vi "Process.vi"(9 "process sync":refnum<notifier>, 11 "Log_Engine in":refnum<class "Log_Engine.lvclass">) -> ()   [LabVIEW 2019, in "Log_Engine.lvclass"]
doc: "Developed by Kevin Thompson\nkevin@thompsonengineering.net\n\nCopyright 2018\nThompson Engineering, LLC"
uses:
  Log_Engine.lvclass
  DataTypes/Read Data--cluster.ctl
  DataTypes/AsynCmd_Log_Engine--enum.ctl
  DataTypes/Process - AppData--cluster.ctl
  DataTypes/Settings--cluster.ctl
  DataTypes/Dependency--cluster.ctl
  Config/Config.lvclass
  DAQ_Engine/DAQ_Engine.lvclass
  DataTypes/Public Events--cluster.ctl
  Common/DataTypes/TD Async CmdMsg EventData--cluster.ctl
  DataTypes/LogStateChg EvData--cluster.ctl
  DataTypes/LogStateEvData--cluster.ctl
  Common/DataTypes/LogState--enum.ctl
  DataTypes/TDMSStateChg EvData--cluster.ctl
  DataTypes/TDMSStateEvData--cluster.ctl
  Common/DataTypes/TDMSState--enum.ctl
  Common/DataTypes/InverterWaveforms--QRef.ctl
  Common/DataTypes/InverterWaveforms--cluster.ctl
  Common/DataTypes/ChannelWaveforms--cluster.ctl
  DataTypes/WriteLoopPvtData--Cluster.ctl
  Log_Engine.lvclass/Log_Engine.ctl
  DAQ_Engine/DAQ_Engine.lvclass/DAQ_Engine.ctl
  Accessors/Get Settings.vi
  Accessors/Get PublicEvents.vi
  Accessors/Get Dependency.vi
  Accessors/Get InvWfmsQRef.vi
  <vilib>/TELLC/SMQ/Add States to Queue using MultiLine String with vData.vi
  <userlib>/_OpenG.lib/file/file.llb/File Exists - Scalar__ogtk.vi
  <vilib>/Utility/file.llb/Write Delimited Spreadsheet (string).vi
panel:
  out "Log_Engine ReadData":T1
  in  "Exit":bool
  # "local data monitoring"
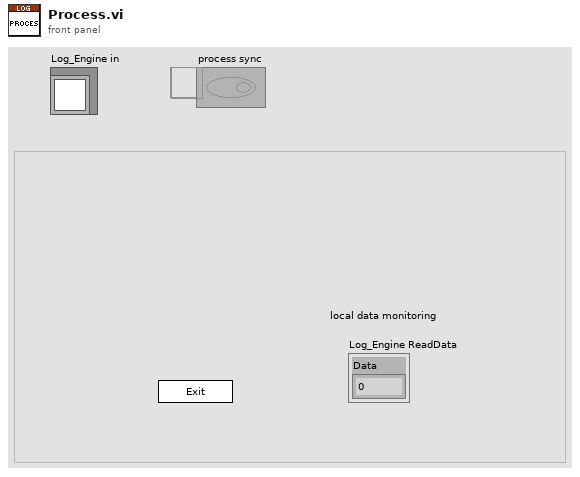
[diagram p1: front panel]
types:
  T1 = typedef "Log_Engine.lvclass/Read Data--cluster.ctl" = cluster{"Data":dbl}
  T2 = typedef "Log_Engine.lvclass/AsynCmd_Log_Engine--enum.ctl" = enum16{"Log_Engine.StartLog", "Log_Engine.StopLog", "Log_Engine.StartESRLog", "Log_Engine.StopESRLog"}
  T3 = typedef "InverterWaveforms--QRef.ctl" = refnum<queue>
  T4 = typedef "InverterWaveforms--cluster.ctl" = cluster{"Phase1 ChanWfms":T5, "Phase2 ChanWfms":T5, "Phase3 ChanWfms":T5}
  T5 = typedef "ChannelWaveforms--cluster.ctl" = cluster{"Iin ripple ":waveform(dbl), "Iout ripple ":waveform(dbl), "Vout 60Hz":waveform(dbl), "Iout 60Hz":waveform(dbl)}
  T6 = typedef "TD MeasData--cluster.ctl" = cluster{"Timestamp":timestamp, "ESR_Ohm":dbl[], "DUT data":T7[], "DUT INVERTER data":cluster{"Raw ESR sum":dbl, "scaled raw ESR sum":dbl, "scaled and averaged raw ESR sum":dbl, "Total power":dbl}[]}
  T7 = typedef "InverterPhaseData--cluster.ctl" = cluster{"RawESR_Ohm":dbl, "TcompAvgESR_Ohm":dbl, "VoutRMS_V":dbl, "IoutRMS_A":dbl, "PF":dbl, "AvgPF":dbl, "Power_W":dbl, "AvgPower_W":dbl, "efficiency":dbl}
  T8 = typedef "Log_Engine.lvclass/Process - AppData--cluster.ctl" = cluster{"Core":cluster{"Current VI Reference":refnum<vi>, "Close Panel on Exit?":bool}, "Your Boolean data":bool, "Your string data":string, "SMQ":refnum<queue>, "Self Reference":refnum<class "Log_Engine.lvclass">, "Simulation?":bool, "process sync":refnum<notifier>, "vData":variant, "Settings":T9, "Dependency":T10, "Public Events":T11, "InverterWaveformsQ":T3, "FileHandle":T12, "Initialized?":bool, "LogState":T13, "TDMSState":T14, "CSV BaseFN":string[], "TDMS BaseFN":string[], "TDMS_Folder":path, "CSV_Folder":path}
  T9 = typedef "Log_Engine.lvclass/Settings--cluster.ctl" = cluster{"Simulation":bool, "TDMS_FolderPath":string, "CSV_FolderPath":string, "TDMS_FileName_Prefix":string, "CSV_FileName_Prefix":string, "TDMS_LogDuration(s)":dbl, "CSV_LogDuration(s)":dbl}
  T10 = typedef "Log_Engine.lvclass/Dependency--cluster.ctl" = cluster{"Config":refnum<class "Config.lvclass">, "DAQ_Engine":refnum<class "DAQ_Engine.lvclass">}
  T11 = typedef "Log_Engine.lvclass/Public Events--cluster.ctl" = cluster{"Log_Engine.AsyncCmd Event":refnum<user-event>, "Log_Engine.AsyncMsg Event":refnum<user-event>, "stop process":refnum<user-event>, "Log_Engine.LogStateChg Ev":refnum<user-event>, "Log_Engine.TDMSStateChg Ev":refnum<user-event>}
  T12 = typedef "Log_Engine.lvclass/WriteLoopPvtData--Cluster.ctl" = cluster{"CSV File Path":path[], "CSV_Initialized":bool, "tdms file ref":refnum<k34>[], "tdms_Initialized":bool, "TDMS File Start Time":dbl, "CSV File Start Time":dbl, "TDMSFileCounter":u32, "CSVFileCounter":u32}
  T13 = typedef "LogState--enum.ctl" = enum16{"Unknown", "Stopped", "Running", "Error"}
  T14 = typedef "TDMSState--enum.ctl" = enum16{"Unknown", "Stopped", "Running", "Error"}
  T15 = enum16{"open", "open or create", "create or replace", "create", "open (read-only)"}
  T16 = enum16{"open", "replace", "create", "open or create", "replace or create", "replace or create with confirmation"}
  T17 = typedef "TD Pathnames--cluster.ctl" = cluster{"RunTimeSys?":bool, "AppFolder":path, "ExecutablePath":path, "ConfigFolder":path, "DataLogFolder":path, "SystemLogFolder":path, "SeqFolder":path, "MainStartupPathname":path, "MainUIPathname":path, "SystemEventsFile":path, "SeqEventsFile":path, "Config SettingsFile":path, "DAQ IOConfigFile":path, "SystemSimulation":bool}
  T18 = typedef "InverterWaveforms--cluster.ctl" = T5[]
  T19 = enum32{"invalid app kind", "Development System", "Run Time System", "Student Edition", "Embedded LabVIEW", "Evaluation", "Custom"}
  T20 = enum32{"Invalid", "Standard", "Closed", "Hidden", "Minimized", "Maximized"}
  T21 = typedef "DAQ_Engine.lvclass/DAQStateEvData--cluster.ctl" = cluster{"DAQState":T22, "vData":variant}
  T22 = typedef "DAQState--enum.ctl" = enum16{"Unknown", "Stopped", "Running", "Error"}
  T23 = cluster{"Current VI Reference":refnum<vi>, "Close Panel on Exit?":bool}
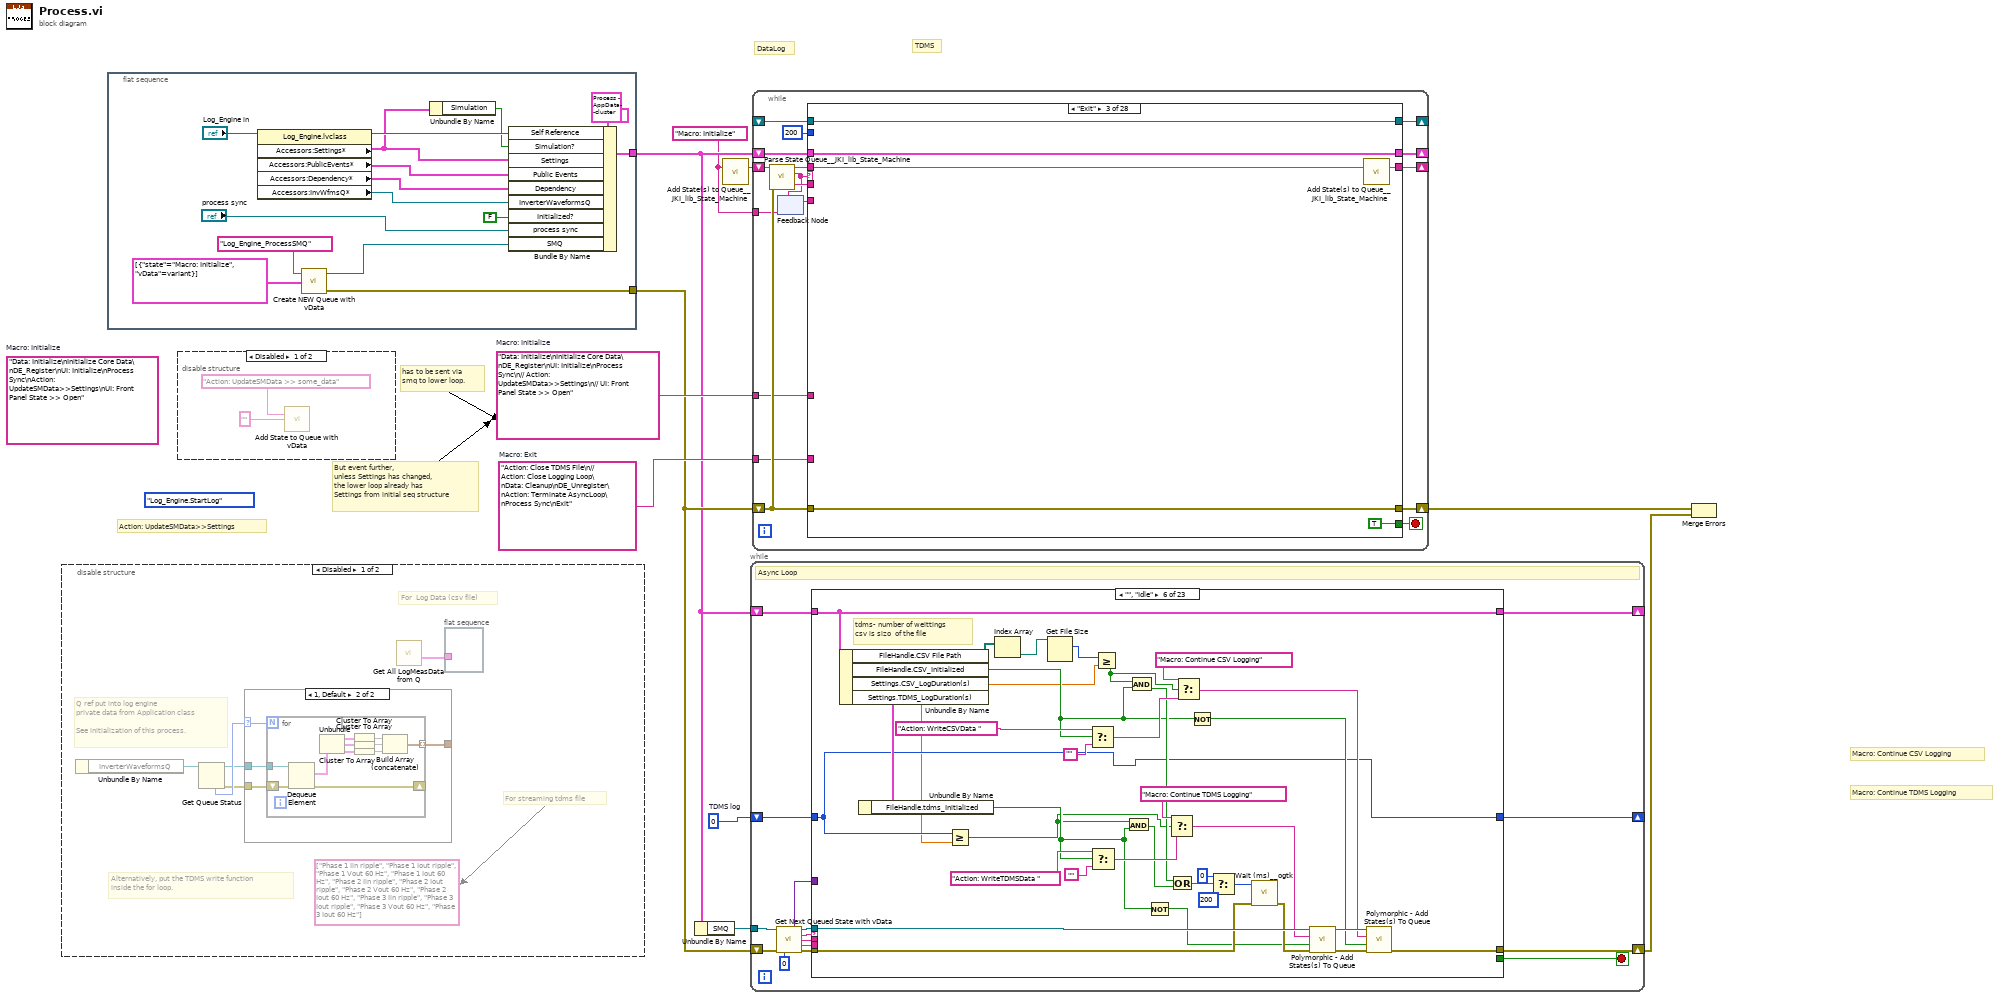
[diagram p0: block diagram]
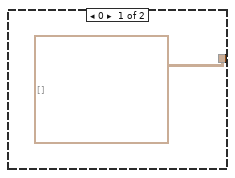
[diagram p2: hidden frame]
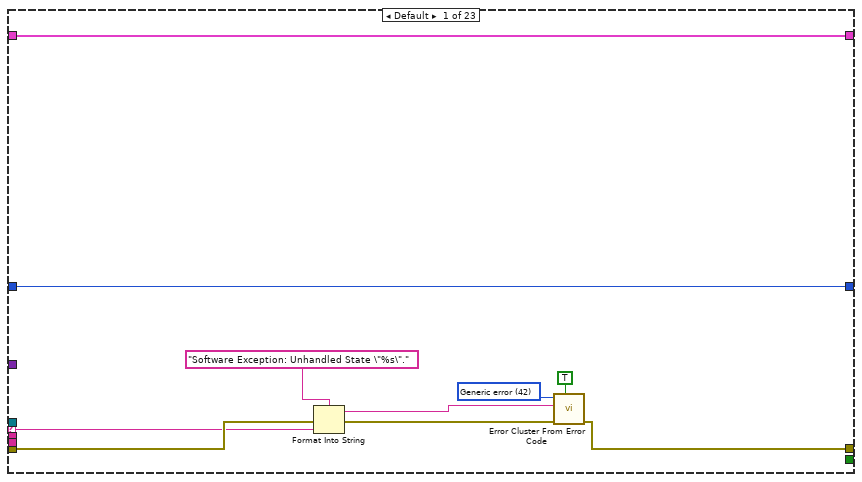
[diagram p5: hidden frame]
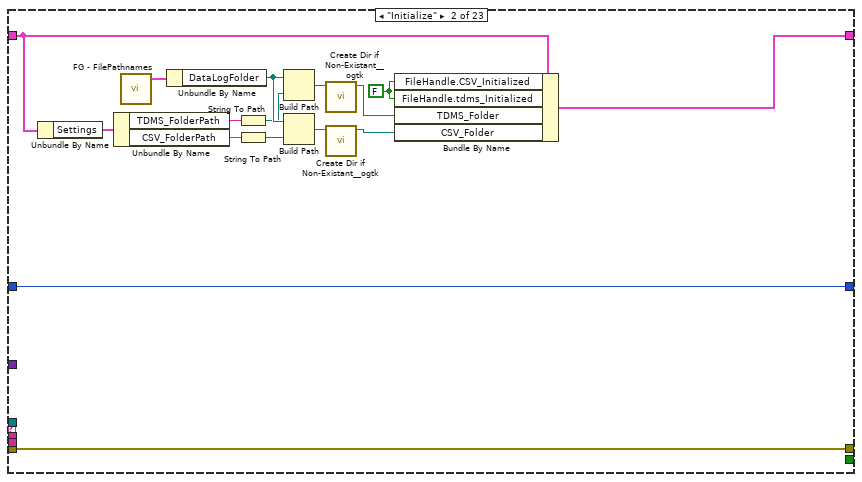
[diagram p6: hidden frame]
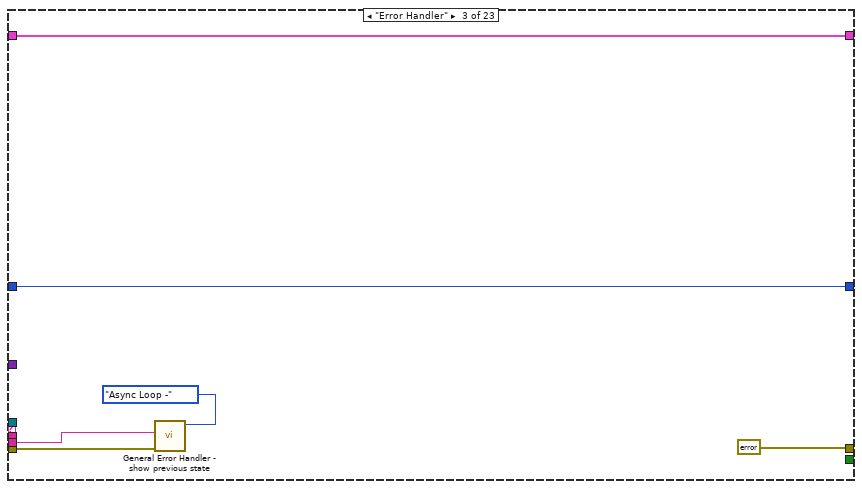
[diagram p7: hidden frame]
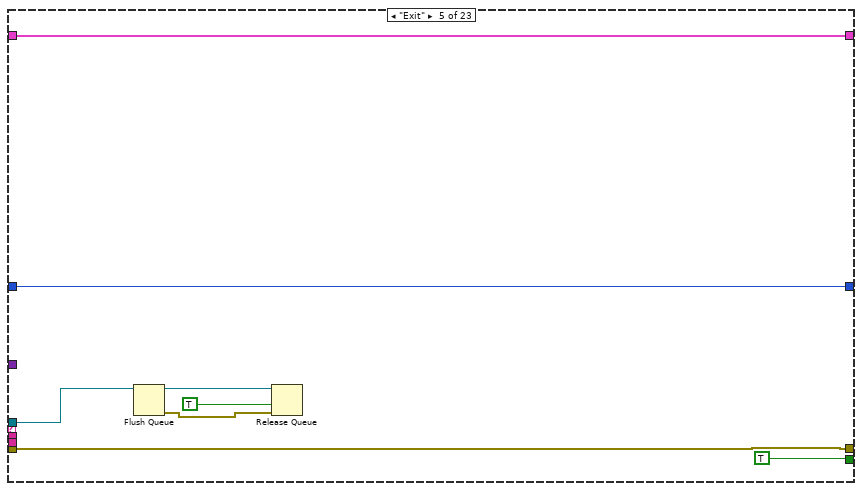
[diagram p9: hidden frame]
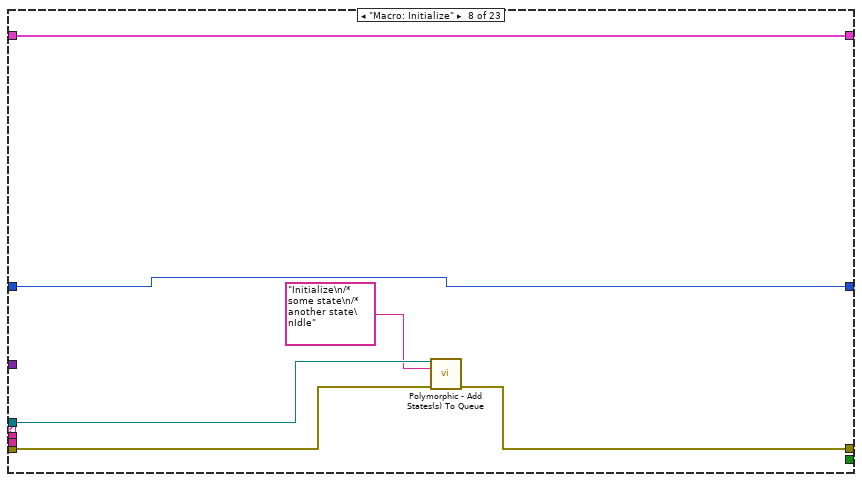
[diagram p11: hidden frame]
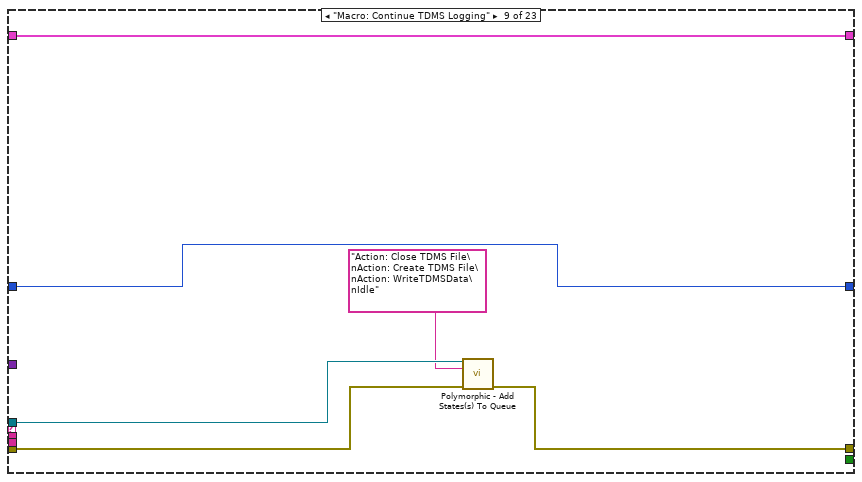
[diagram p12: hidden frame]
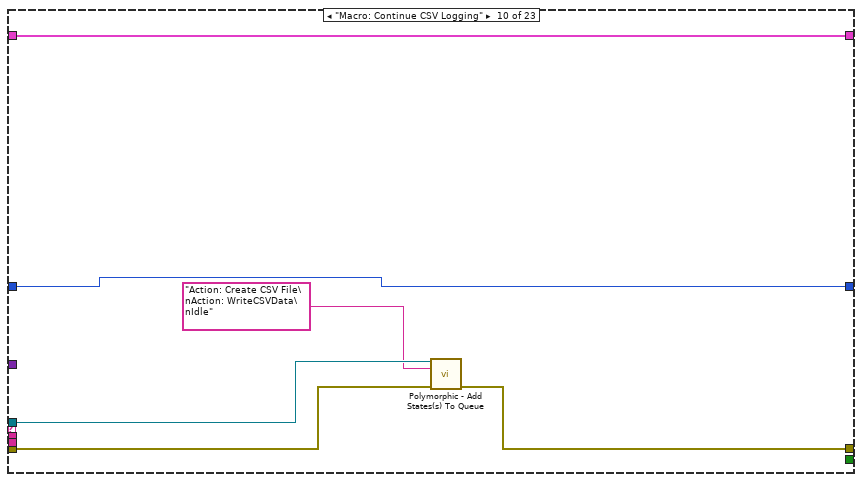
[diagram p13: hidden frame]
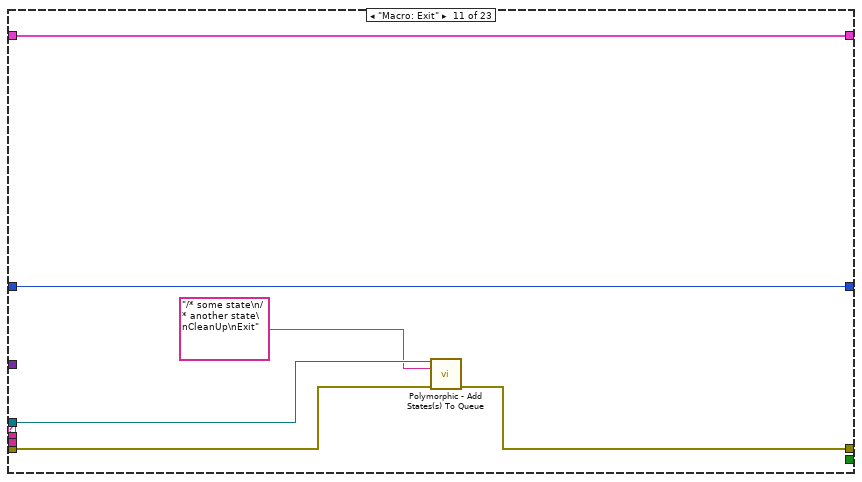
[diagram p14: hidden frame]
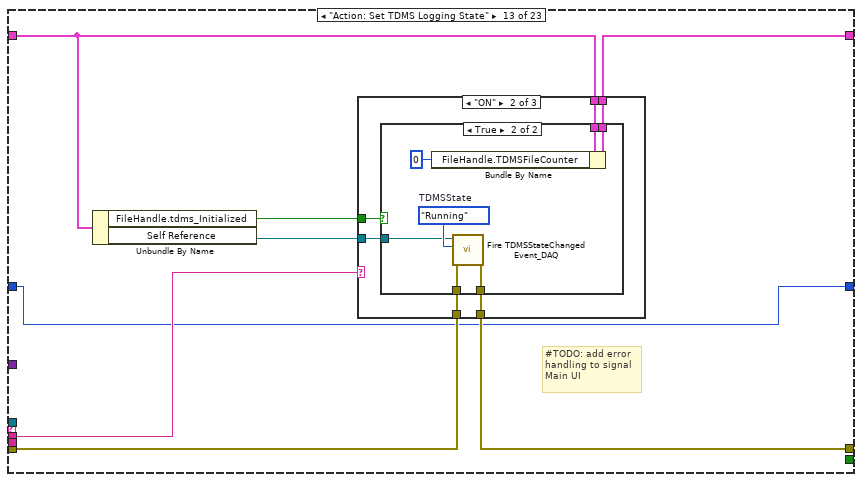
[diagram p16: hidden frame]
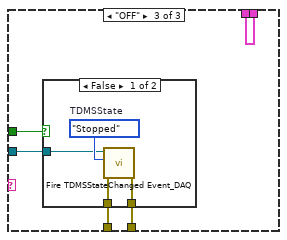
[diagram p19: hidden frame]
diagram:
  w1 = 0  # TDMS log
  (unwired) "Data: Initialize\nInitialize Core Data\nDE_Register\nUI: Initialize\nProcess Sync\nAction: UpdateSMData>>Settings\nUI: Front Panel State >> Open"  # Macro: Initialize
  (unwired) AsynCmd_Log_Engine--enum."Log_Engine.StartLog" ("AsyncCmd")
  w8 = "Action: Close TDMS File\n// Action: Close Logging Loop\nData: Cleanup\nDE_Unregister\nAction: Terminate AsyncLoop\nProcess Sync\nExit"  # Macro: Exit
  w9 = "Data: Initialize\nInitialize Core Data\nDE_Register\nUI: Initialize\nProcess Sync\n// Action: UpdateSMData>>Settings\n// UI: Front Panel State >> Open"  # Macro: Initialize
  w2 = "Macro: Initialize"
  # "TDMS"
  # "DataLog"
  # "Macro: Continue TDMS Logging"
  # "Macro: Continue CSV Logging"
  # "But event further,\nunless Settings has changed,\nthe lower loop already has\nSettings from initial seq structure"
  # "has to be sent via\nsmq to lower loop."
  # "Action: UpdateSMData>>Settings"
  n1 = disable-structure shown="Disabled" {
    frame Disabled {
      (unwired) string[] ["Phase 1 Iin ripple", "Phase 1 Iout ripple", "Phase 1 Vout 60 Hz", "Phase 1 Iout 60 Hz", "Phase 2 Iin ripple", "Phase 2 Iout ripple", "Phase 2 Vout 60 Hz", "Phase 2 Iout 60 Hz", "Phase 3 Iin ripple", "Phase 3 Iout ripple", "Phase 3 Vout 60 Hz", "Phase 3 Iout 60 Hz"] ("channel name(s) in (Untitled)")
      # "Q ref put into log engine\nprivate data from Application class\n\nSee initialization of this process."
      # "Alternatively, put the TDMS write function\ninside the for loop."
      # "For streaming tdms file"
      # "For  Log Data (csv file)"
      n2 = Unbundle By Name() -> ("InverterWaveformsQ"=w11:T3)  [unwired: 1 in]
      n3 = Get Queue Status(queue=w11) -> (queue out=w14:T3, error out=w13:errorcluster, # elements in queue=w15:i32)  [unwired: 2 in, 5 out]
      n4 = case shown="1, Default" w15 {
        selector: w15 -> [_ w20]
        tunnel: w14 -> [_ w19]
        tunnel: w13 -> [_ w18]
        tunnel: [waveform(dbl)[][] [] w17] -> _
        frame 0 {
        }
        frame 1, Default {
          n5 = for {
            N: w20 -> [_]
            tunnel: w19 -> [w31]
            shift-right: [w29] -> _
            shift-left: w18 -> [w30]
            tunnel: [w21] -> w17 mode=indexing
            n6 = Dequeue Element(queue=w31, error in (no error)=w30) -> (element=w28:T4, error out=w29:errorcluster)  [unwired: 1 in, 2 out]
            n7 = Unbundle(w28) -> ("Phase1 ChanWfms"=w27:T5, "Phase2 ChanWfms"=w26:T5, "Phase3 ChanWfms"=w25:T5)
            n8 = Cluster To Array(cluster=w27) -> (array=w24:waveform(dbl)[])
            n9 = Cluster To Array(cluster=w26) -> (array=w23:waveform(dbl)[])
            n10 = Cluster To Array(cluster=w25) -> (array=w22:waveform(dbl)[])
            n11 = Build Array (concatenate)(w24, w23, w22) -> (w21:waveform(dbl)[])
          }
        }
      }
      n12 = call "Get All LogMeasData from Q.vi"() -> ("MeasData[] out"=w12:T6[])  [unwired: 8 in, 3 out]
      n13 = flat-sequence {
        tunnel: w12 -> [_]
        frame #0 {
        }
      }
    }
    frame Enabled {
    }
  }
  n14 = flat-sequence {
    tunnel: [w46] -> w5
    tunnel: [w43] -> w7
    frame #0 {
      n15 = property class="Log_Engine.lvclass"(reference="Log_Engine in") -> (reference out=w40:refnum<class "Log_Engine.lvclass">, "Accessors:Settings*"=w32:T9, "Accessors:PublicEvents*"=w37:T11, "Accessors:Dependency*"=w38:T10, "Accessors:InvWfmsQ*"=w34:T3)  [unwired: 1 in, 1 out]
      n16 = call <vilib>:"Create NEW Queue with vData.vi"("Initial States"=cluster{"state":string, "vData":variant}[] [{"state"="Macro: Initialize", "vData"=variant}], "Name (SMQ)"="Log_Engine_ProcessSMQ") -> ("error out"=w43:errorcluster, "queue out"=w45:refnum<queue>)  [unwired: 2 in]
      n17 = Unbundle By Name(w32) -> ("Simulation"=w33:bool)
      n18 = Bundle By Name(cluster=T8 {"Core"={"Current VI Reference"=refnum, "Close Panel on Exit?"=FALSE}, "Your Boolean data"=FALSE, "Your string data"="", "SMQ"=refnum, "Self Reference"=refnum, "Simulation?"=FALSE, "process sync"=refnum, "vData"=variant, "Settings"={"Simulation"=FALSE, "TDMS_FolderPath"="", "CSV_FolderPath"="", "TDMS_FileName_Prefix"="", "CSV_FileName_Prefix"="", "TDMS_LogDuration(s)"=0.0, "CSV_LogDuration(s)"=0.0}, "Dependency"={"Config"=refnum, "DAQ_Engine"=refnum}, "Public Events"={"Log_Engine.AsyncCmd Event"=refnum, "Log_Engine.AsyncMsg Event"=refnum, "stop process"=refnum, "Log_Engine.LogStateChg Ev"=refnum, "Log_Engine.TDMSStateChg Ev"=refnum}, "InverterWaveformsQ"=refnum, "FileHandle"={"CSV File Path"=[], "CSV_Initialized"=FALSE, "tdms file ref"=[], "tdms_Initialized"=FALSE, "TDMS File Start Time"=0.0, "CSV File Start Time"=0.0, "TDMSFileCounter"=0, "CSVFileCounter"=0}, "Initialized?"=FALSE, "LogState"=enum."Unknown", "TDMSState"=enum."Unknown", "CSV BaseFN"=[], "TDMS BaseFN"=[], "TDMS_Folder"=path "", "CSV_Folder"=path ""} ("SM2 AppData"), "Self Reference"=w40, "Simulation?"=w33, "Settings"=w32, "Public Events"=w37, "Dependency"=w38, "InverterWaveformsQ"=w34, "Initialized?"=FALSE, "process sync"="process sync", "SMQ"=w45) -> (w46:T8)
    }
  }
  n19 = disable-structure shown="Disabled" {
    frame Disabled {
      n20 = call <vilib>:"Add State to Queue with vData.vi"("state in"="Action: UpdateSMData >> some_data", "vData (\"\")"="") -> ()  [unwired: 10 in, 4 out]
    }
    frame Enabled {
    }
  }
  n21 = Unbundle By Name(w5) -> ("SMQ"=w6:refnum<queue>)
  n22 = call <vilib>:"Add State(s) to Queue__JKI_lib_State_Machine.vi"("State(s) in (\"\")"=w2) -> ("States Out"=w10:string)  [unwired: 14 in]
  n23 = while {
    shift-right: [w60] -> w3
    shift-left: w7 -> [w62]
    tunnel: w6 -> [w58]
    shift-right: [w56] -> _
    shift-left: w5 -> [w57]
    shift-right: [w50] -> _
    shift-left: w1 -> [w49]
    stop <- w51 stop-if-true
    # "Async Loop"
    n24 = call <vilib>:"Get Next Queued State with vData.vi"("queue in"=w58, "error in (no error)"=w62, "timeout (100)"=0) -> ("vData out"=w55:variant, "queue out"=w59:refnum<queue>, "Next State"=w63:string, "queued msg"=w53:string, "Prev State"=w52:string, "error out"=w61:errorcluster)  [unwired: 6 in, 1 out]
    n25 = case shown="\"\", \"Idle\"" w63 {
      tunnel: w59 -> [_ _ _ _ w100 w134 _ w149 w155 w161 w167 _ _ _ _ _ _ _ _ _ _ _ w398]
      tunnel: w53 -> [_ _ _ _ _ _ _ _ _ _ _ _ w178 w213 _ _ _ _ _ _ _ w386 w400]
      selector: w63 -> [w65 _ _ _ _ _ _ _ _ _ _ _ _ _ _ _ _ _ _ _ _ _ _]
      tunnel: w61 -> [w67 w89 w92 w98 w106 w126 w144 w148 w154 w160 w166 w171 w175 w210 w243 w270 w312 w343 w361 w373 w380 w385 w395]
      tunnel: [w66 w89 errorcluster {"status"=FALSE, "code"=0, "source"=""} ("error constant") w98 w106 w133 w144 w147 w153 w159 w165 w171 w176 w211 w252 w277 w314 w340 w357 w373 w379 w388 w394] -> w60
      tunnel: w57 -> [w73 w85 w95 w97 w105 w135 w143 w150 w156 w162 w168 w170 w173 w208 w256 w281 w311 w344 w359 w374 w382 w391 w397]
      tunnel: [w73 w87 w95 w97 w105 w135 w143 w150 w156 w162 w168 w170 w174 w209 w259 w287 w311 w344 w358 w376 w382 w391 w396] -> w56
      tunnel: w55 -> [_ _ _ _ _ _ _ _ _ _ _ _ _ _ _ _ _ _ _ _ _ _ w399]
      tunnel: w52 -> [_ _ w91 _ _ _ _ _ _ _ _ _ _ _ _ _ _ _ _ _ _ _ _]
      tunnel: [_ _ _ _ TRUE _ _ _ _ _ _ _ _ _ _ _ _ _ _ _ _ _ _] -> w51
      tunnel: [w64 w74 w90 w96 w99 w114 w142 w145 w151 w157 w163 w169 w172 w207 0 w276 w309 w338 w356 w372 w377 w383 w392] -> w50
      tunnel: w49 -> [w64 w74 w90 w96 w99 w114 w142 w145 w151 w157 w163 w169 w172 w207 _ w276 w310 w338 w356 w372 w377 w383 w392]
      frame Default {
        w69 = 42 items=["No error", "Argument error", "Memory is full", "Out of zone", "End of file", "File already open", "Generic file I/O error", "File not found", "File permission error", "Disk is full", "Duplicate path", "Too many files open", "System feature not enabled", "Resource file not found", "Cannot add resource", "Resource not found", "Image not found", "Image memory error", "Pen does not exist", "Config type invalid", "Config token not found", "Config parse error", "Config memory error", "Bad external code format", "Bad external code offset", "External code not present", "Null window", "Destroy window error", "Null menu", "Print aborted", "Bad print record", "Print driver error", "Windows error during printing", "Memory error during printing", "Print dialog error", "Generic print error", "Invalid device refnum", "Device not found", "Device parameter error", "Device unit error", "Cannot open device", "Device call aborted", "Generic error", "Cancelled by user", "Object ID too low", "Object ID too high", "Object not in heap", "Unknown heap", "Unknown object (invalid DefProc)", "Unknown object (DefProc not in table)", "Message out of range", "Invalid (null) method", "Unknown message", "Manager call not supported", "Bad address", "Network operation in progress", "Network operation timed out", "Connection is busy", "Network attribute not supported", "Network error", "Address in use", "System out of memory", "Connection aborted", "Connection refused", "Not connected", "Already connected", "Connection closed", "Initialization error (interapplication manager)", "Bad occurrence", "Wait on unbound occurrence handler", "Occurrence queue overflow", "Datalog type conflict", "Unused", "Unrecognized type (interapplication manager)", "Memory corrupt", "Failed to make temporary DLL", "Old CIN version", "Drag socket not found", "Failed to load drop-object", "Failed to register OLE object", "Failed to release OLE object", "Format specifier type mismatch", "Unknown format specifier", "Too few format specifiers", "Too many format specifiers", "Scan failed", "Newer CIN version", "Error converting to variant", "Runtime menu error", "Password tampered", "Variant attribute not found", "Incompatible variant data type", "Event data is not available", "Event Store is not present", "Occurrence is not found", "Event Queue is not created", "Event info is not available", "Refnum passed is NULL", "Error retrieving Class GUID", "Error retrieving CoClass GUID", "Error retrieving TypeLib GUID.", "Bad built application magic bytes.", "Specific driver is different from the specific driver associated with the Logical Name.", "There is no session opened to the class driver.", "Max Error", "MAX - Error with config objects", "MAX - Error loading configuration", "MAX - Group not supported"]
        n26 = Format Into String(format string="Software Exception: Unhandled State \"%s\"." ("message"), error in=w67, w65) -> (resulting string=w70:string, error out=w71:errorcluster)  [unwired: 1 in]
        n27 = call <vilib>:"Error Cluster From Error Code.vi"("show call chain? (False)"=TRUE, "error in (no error)"=w71, "error message (\"\")"=w70, "error code (0)"=w69) -> ("error out"=w66:errorcluster)  [unwired: 5 in]
      }
      frame "Initialize" {
        w88 = FALSE
        n28 = Unbundle By Name(w85) -> ("Settings"=w84:T9)
        n29 = Unbundle By Name(w84) -> ("TDMS_FolderPath"=w80:string, "CSV_FolderPath"=w79:string)
        n30 = call "FG - FilePathnames.vi"() -> ("FilePaths out"=w83:T17)  [unwired: 4 in, 1 out]
        n31 = Unbundle By Name(w83) -> ("DataLogFolder"=w82:path)
        n32 = String To Path(string=w80) -> (path=w78:path)
        n33 = String To Path(string=w79) -> (path=w77:path)
        n34 = Build Path(base path=w82, name or relative path=w78) -> (appended path=w76:path)
        n35 = Build Path(base path=w82, name or relative path=w77) -> (appended path=w75:path)
        n36 = call <userlib>:"Create Dir if Non-Existant__ogtk.vi"("Directory Path"=w76) -> ("dup Directory Path"=w81:path)  [unwired: 8 in, 2 out]
        n37 = call <userlib>:"Create Dir if Non-Existant__ogtk.vi"("Directory Path"=w75) -> ("dup Directory Path"=w86:path)  [unwired: 8 in, 2 out]
        n38 = Bundle By Name(cluster=w85, "FileHandle.CSV_Initialized"=w88, "FileHandle.tdms_Initialized"=w88, "TDMS_Folder"=w81, "CSV_Folder"=w86) -> (w87:T8)
      }
      frame "Error Handler" {
        n39 = call "General Error Handler - show previous state.vi"("error in (no error)"=w92, "Previous State"=w91, "Loop Select"=enum16{"Event Loop -", "Async Loop -"}."Async Loop -") -> ()  [unwired: 7 in, 2 out]
      }
      frame "CleanUp" {
      }
      frame "Exit" {
        n40 = Flush Queue(queue=w100) -> (queue out=w103:refnum<queue>, error out=w102:errorcluster)  [unwired: 1 in, 1 out]
        n41 = Release Queue(queue=w103, force destroy? (F)=TRUE, error in (no error)=w102) -> ()  [unwired: 3 out]
      }
      frame "", "Idle" {
        # "tdms- number of weittings\ncsv is sizo  of the file"
        n42 = Unbundle By Name(w135) -> ("FileHandle.CSV File Path"=w112:path[], "FileHandle.CSV_Initialized"=w118:bool, "Settings.CSV_LogDuration(s)"=w108:dbl, "Settings.TDMS_LogDuration(s)"=w107:dbl)
        n43 = Unbundle By Name(w135) -> ("FileHandle.tdms_Initialized"=w116:bool)
        n44 = Greater Or Equal?(x=w114, y=w107) -> (x >= y?=w113:bool)
        n45 = Index Array(array=w112) -> (element=w111:path)  [unwired: 1 in]
        n46 = Get File Size(file=w111) -> (size (in bytes)=w110:i64)  [unwired: 1 in, 2 out]
        n47 = Select(t="Action: WriteCSVData ", s=w118, f="") -> (s? t:f=w139:string)
        n48 = Select(t="Action: WriteTDMSData ", s=w116, f="") -> (s? t:f=w138:string)
        n49 = Greater Or Equal?(x=w110, y=w108) -> (x >= y?=w109:bool)
        n50 = And(x=w113, y=w116) -> (x .and. y?=w128:bool)
        n51 = And(x=w109, y=w118) -> (x .and. y?=w127:bool)
        n52 = Not(x=w116) -> (.not. x?=w115:bool)
        n53 = Select(t="Macro: Continue TDMS Logging", s=w113, f=w138) -> (s? t:f=w123:string)
        n54 = Or(x=w127, y=w128) -> (x .or. y?=w129:bool)
        n55 = Select(t="Macro: Continue CSV Logging", s=w109, f=w139) -> (s? t:f=w121:string)
        n56 = Not(x=w118) -> (.not. x?=w117:bool)
        n57 = Select(t=u32 0, s=w129, f=u32 200) -> (s? t:f=w132:u32)
        n58 = call <userlib>:"Wait (ms)__ogtk.vi"("error in (no error)"=w126, "milliseconds to wait"=w132) -> ("error out"=w124:errorcluster)  [unwired: 8 in, 1 out]
        n59 = call-poly <vilib>:"Polymorphic - Add States(s) To Queue.vi"("queue in"=w134, "state in"=w123, "bypass (F)"=w115, "error in"=w124) -> ("queue out"=w125:refnum<queue>, "error out"=w122:errorcluster)  [unwired: 8 in, 2 out]
        n60 = call-poly <vilib>:"Polymorphic - Add States(s) To Queue.vi"("queue in"=w125, "state in"=w121, "bypass (F)"=w117, "error in"=w122) -> ("error out"=w133:errorcluster)  [unwired: 8 in, 3 out]
      }
      frame "------ Macro ------" {
      }
      frame "Macro: Initialize" {
        n61 = call-poly <vilib>:"Polymorphic - Add States(s) To Queue.vi"("queue in"=w149, "states in"="Initialize\n/* some state\n/* another state\nIdle", "error in"=w148) -> ("error out"=w147:errorcluster)  [unwired: 10 in, 2 out]
      }
      frame "Macro: Continue TDMS Logging" {
        n62 = call-poly <vilib>:"Polymorphic - Add States(s) To Queue.vi"("queue in"=w155, "states in"="Action: Close TDMS File\nAction: Create TDMS File\nAction: WriteTDMSData\nIdle", "error in"=w154) -> ("error out"=w153:errorcluster)  [unwired: 10 in, 2 out]
      }
      frame "Macro: Continue CSV Logging" {
        n63 = call-poly <vilib>:"Polymorphic - Add States(s) To Queue.vi"("queue in"=w161, "states in"="Action: Create CSV File\nAction: WriteCSVData\nIdle", "error in"=w160) -> ("error out"=w159:errorcluster)  [unwired: 10 in, 2 out]
      }
      frame "Macro: Exit" {
        n64 = call-poly <vilib>:"Polymorphic - Add States(s) To Queue.vi"("queue in"=w167, "states in"="/* some state\n/* another state\nCleanUp\nExit", "error in"=w166) -> ("error out"=w165:errorcluster)  [unwired: 10 in, 2 out]
      }
      frame "------ Action ------" {
      }
      frame "Action: Set TDMS Logging State" {
        # "#TODO: add error\nhandling to signal\nMain UI"
        n65 = Unbundle By Name(w173) -> ("FileHandle.tdms_Initialized"=w177:bool, "Self Reference"=w179:refnum<class "Log_Engine.lvclass">)
        n66 = case shown="\"ON\"" w178 {
          tunnel: w179 -> [_ w186 w200]
          tunnel: w177 -> [_ w187 w201]
          tunnel: w175 -> [w181 w185 w199]
          tunnel: [w181 w184 w198] -> w176
          tunnel: w173 -> [w180 w183 w197]
          tunnel: [w180 w182 w197] -> w174
          frame "False", Default {
            # "#TODO: add error\nhandling to signal\nMain UI"
          }
          frame "ON" {
            n67 = case shown="True" w187 {
              tunnel: w186 -> [_ w195]
              tunnel: w185 -> [w189 w194]
              tunnel: [w189 w193] -> w184
              tunnel: w183 -> [w188 w192]
              tunnel: [w188 w191] -> w182
              frame False {
                # "#TODO: add error\nhandling to signal\nMain UI"
              }
              frame True {
                w196 = TDMSState--enum."Running"  # TDMSState
                n68 = Bundle By Name(cluster=w192, "FileHandle.TDMSFileCounter"=u32 0) -> (w191:T8)
                n69 = call "Fire TDMSStateChanged Event_DAQ.vi"("error in (no error)"=w194, "DAQState"=w196, "Log_Engine in"=w195) -> ("error out"=w193:errorcluster)  [unwired: 7 in, 1 out]
              }
            }
          }
          frame "OFF" {
            n70 = case shown="False" w201 {
              tunnel: w200 -> [w204 _]
              tunnel: w199 -> [w203 w206]
              tunnel: [w202 w206] -> w198
              frame False {
                w205 = TDMSState--enum."Stopped"  # TDMSState
                n71 = call "Fire TDMSStateChanged Event_DAQ.vi"("error in (no error)"=w203, "DAQState"=w205, "Log_Engine in"=w204) -> ("error out"=w202:errorcluster)  [unwired: 7 in, 1 out]
              }
              frame True {
                # "#TODO: add error\nhandling to signal\nMain UI"
              }
            }
          }
        }
      }
      frame "Action: Set CSV Logging State" {
        # "#TODO: add error\nhandling to signal\nMain UI"
        n72 = Unbundle By Name(w208) -> ("FileHandle.CSV_Initialized"=w212:bool, "Self Reference"=w214:refnum<class "Log_Engine.lvclass">)
        n73 = case shown="\"ON\"" w213 {
          tunnel: w214 -> [_ w221 w235]
          tunnel: w212 -> [_ w222 w236]
          tunnel: w210 -> [w216 w220 w234]
          tunnel: [w216 w219 w233] -> w211
          tunnel: w208 -> [w215 w218 w232]
          tunnel: [w215 w217 w232] -> w209
          frame "False", Default {
            # "#TODO: add error\nhandling to signal\nMain UI"
          }
          frame "ON" {
            n74 = case shown="True" w222 {
              tunnel: w221 -> [_ w231]
              tunnel: w220 -> [w224 w230]
              tunnel: [w224 w229] -> w219
              tunnel: w218 -> [w223 w228]
              tunnel: [w223 w227] -> w217
              frame False {
                # "#TODO: add error\nhandling to signal\nMain UI"
              }
              frame True {
                w225 = LogState--enum."Running"  # LogState
                n75 = Bundle By Name(cluster=w228, "FileHandle.CSVFileCounter"=u32 0 ("FileHandle.TDMSFileCounter")) -> (w227:T8)
                n76 = call "Fire LogStateChanged Event_DAQ.vi"("error in (no error)"=w230, "DAQState"=w225, "Log_Engine in"=w231) -> ("error out"=w229:errorcluster)  [unwired: 7 in, 1 out]
              }
            }
          }
          frame "OFF" {
            n77 = case shown="False" w236 {
              tunnel: w235 -> [w240 _]
              tunnel: w234 -> [w239 w241]
              tunnel: [w238 w241] -> w233
              frame False {
                w237 = LogState--enum."Stopped"  # LogState
                n78 = call "Fire LogStateChanged Event_DAQ.vi"("error in (no error)"=w239, "DAQState"=w237, "Log_Engine in"=w240) -> ("error out"=w238:errorcluster)  [unwired: 7 in, 1 out]
              }
              frame True {
                # "#TODO: add error\nhandling to signal\nMain UI"
              }
            }
          }
        }
      }
      frame "Action: Create TDMS File" {
        n79 = Unbundle By Name(w256) -> ("TDMS_Folder"=w253:path, "FileHandle.TDMSFileCounter"=w246:u32, "Dependency.Config"=w247:refnum<class "Config.lvclass">)
        n80 = call "get inverter SN.vi"("error in"=w243, "File counter"=w246, "Config in"=w247) -> ("error out"=w242:errorcluster, "File namd"=w244:string[], "BaseFN"=w245:string[])  [unwired: 5 in, 1 out]
        n81 = Increment(x=w246) -> (x+1=w249:u32)
        n82 = call <userlib>:"Create Dir if Non-Existant__ogtk.vi"("Directory Path"=w253) -> ("dup Directory Path"=w254:path)  [unwired: 8 in, 2 out]
        n83 = for {
          tunnel: [w268] -> w258 mode=indexing
          tunnel: w254 -> [w266]
          shift-right: [w264] -> w252
          shift-left: w242 -> [w265]
          tunnel: w244 -> [w260] mode=indexing
          n84 = Concatenate Strings(w260, ".tdms" ("string")) -> (w263:string)
          n85 = Build Path(base path=w266, name or relative path=w263) -> (appended path=w267:path)
          n86 = TDMS Open(5:FALSE ("create index file? (T)"), 8:w265, 10:T15."open or create" ("operation (0:open)"), 11:w267) -> (0:w264:errorcluster, 3:w268:refnum<k34>)  [unwired: 3 in]
        }
        n87 = Unbundle By Name(w252) -> ("status"=w255:bool)
        n88 = Get Date/Time In Seconds() -> (seconds since 1Jan1904=w251:timestamp)
        n89 = Not(x=w255) -> (.not. x?=w257:bool)
        n90 = To Double Precision Float(number=w251) -> (double precision float=w250:dbl)
        n91 = Bundle By Name(cluster=w256, "FileHandle.TDMS File Start Time"=w250, "FileHandle.tdms file ref"=w258, "FileHandle.tdms_Initialized"=w257, "FileHandle.TDMSFileCounter"=w249, "TDMS BaseFN"=w245) -> (w259:T8)
      }
      frame "Action: Create CSV File" {
        n92 = Unbundle By Name(w281) -> ("CSV_Folder"=w279:path, "FileHandle.CSVFileCounter"=w272:u32, "Dependency.Config"=w275:refnum<class "Config.lvclass">)  [unwired: 1 out]
        n93 = call "get inverter SN.vi"("error in"=w270, "File counter"=w272, "Config in"=w275) -> ("error out"=w271:errorcluster, "File namd"=w273:string[], "BaseFN"=w274:string[])  [unwired: 5 in, 1 out]
        n94 = call <userlib>:"Create Dir if Non-Existant__ogtk.vi"("Directory Path"=w279) -> ("dup Directory Path"=w278:path)  [unwired: 8 in, 2 out]
        n95 = for {
          tunnel: [w298] -> w285 mode=indexing
          tunnel: w278 -> [w297]
          shift-right: [w294] -> w277
          shift-left: w271 -> [w295]
          tunnel: w273 -> [w289] mode=indexing
          n96 = Concatenate Strings(w289, ".csv" ("string")) -> (w293:string)
          n97 = Build Path(base path=w297, name or relative path=w293) -> (appended path=w296:path)
          n98 = call-poly <userlib>:"File Exists__ogtk.vi"("file path"=w296) -> ("exists"=w299:bool)  [unwired: 6 in, 1 out]
          n99 = case shown="False" w299 {
            tunnel: w296 -> [w301 w307]
            tunnel: [w303 w308] -> w290
            tunnel: w295 -> [w302 w308]
            tunnel: [w301 w307] -> w288
            frame False {
              n100 = Open/Create/Replace File(file path (use dialog)=w301, error in=w302, operation (0:open)=T16."create") -> (refnum out=w305:refnum<file>, error out=w304:errorcluster)  [unwired: 3 in, 1 out]
              n101 = Close File(refnum=w305, error in=w304) -> (error out=w303:errorcluster)  [unwired: 1 out]
            }
            frame True {
            }
          }
          n102 = call "Generate Column Names.vi"() -> ("Names (Array)"=w291:string[])  [unwired: 9 in, 2 out]
          n103 = call-poly <vilib>:"Write Delimited Spreadsheet.vi"("file path (dialog if empty)"=w288, "1D data"=w291, "error in (no error)"=w290, "delimiter (\\t)"="," ("delimiter (\\t)")) -> ("new file path (Not A Path if cancelled)"=w298:path, "error out"=w294:errorcluster)  [unwired: 10 in]
        }
        n104 = Get Date/Time In Seconds() -> (seconds since 1Jan1904=w284:timestamp)
        n105 = Unbundle By Name(w277) -> ("status"=w280:bool)
        n106 = Increment(x=w272) -> (x+1=w282:u32)
        n107 = To Double Precision Float(number=w284) -> (double precision float=w283:dbl)
        n108 = Not(x=w280) -> (.not. x?=w286:bool)
        n109 = Bundle By Name(cluster=w281, "FileHandle.CSV File Start Time"=w283, "FileHandle.CSV_Initialized"=w286, "FileHandle.CSV File Path"=w285, "FileHandle.CSVFileCounter"=w282, "CSV BaseFN"=w274) -> (w287:T8)
      }
      frame "Action: WriteTDMSData" {
        n110 = Unbundle By Name(w311) -> ("FileHandle.tdms file ref"=w316:refnum<k34>[], "Self Reference"=w320:refnum<class "Log_Engine.lvclass">)
        n111 = property class="Log_Engine.lvclass"(reference=w320) -> ("Accessors:InvWfmsQ*"=w317:T3)  [unwired: 1 in, 2 out]
        n112 = Get Queue Status(queue=w317, error in (no error)=w312) -> (queue out=w318:T3, error out=w313:errorcluster, # elements in queue=w319:i32)  [unwired: 1 in, 5 out]
        n113 = case shown="1, Default" w319 {
          tunnel: w318 -> [_ w331]
          tunnel: w313 -> [w322 w330]
          tunnel: w316 -> [_ w329]
          tunnel: string[] ["Iin ripple", "Iout ripple", "Vout 60 Hz", "Iout 60 Hz"] ("channel name(s) in (Untitled)") -> [_ w328]
          tunnel: [w322 w327] -> w314
          tunnel: w310 -> [w321 w324]
          tunnel: [w321 w323] -> w309
          frame 0 {
          }
          frame 1, Default {
            n114 = Dequeue Element(queue=w331, error in (no error)=w330) -> (element=w325:T18, error out=w326:errorcluster)  [unwired: 1 in, 2 out]
            n115 = for {
              tunnel: w328 -> [w337]
              tunnel: w329 -> [w336] mode=indexing
              tunnel: w325 -> [w333] mode=indexing
              shift-right: [w334] -> w327
              shift-left: w326 -> [w335]
              n116 = Cluster To Array(cluster=w333) -> (array=w332:waveform(dbl)[])
              n117 = TDMS Write(0:w336, 7:w337, 9:w332, 11:w335) -> (15:w334:errorcluster)  [unwired: 2 in, 3 out]
            }
            n118 = Increment(x=w324) -> (x+1=w323:i32)
          }
        }
      }
      frame "Action: WriteCSVData" {
        n119 = Unbundle By Name(w344) -> ("FileHandle.CSV File Path"=w339:path[])
        n120 = call "Get All LogMeasData from Q.vi"("error in (no error)"=w343) -> ("error out"=w341:errorcluster, "MeasData[] out"=w342:T6[])  [unwired: 7 in, 2 out]
        n121 = for {
          tunnel: w342 -> [w346] mode=indexing
          shift-right: [w348] -> w340
          shift-left: w341 -> [w349]
          tunnel: w339 -> [w347]
          n122 = call "Generate Column Names.vi"("MeasData"=w346) -> ("Data"=w345:string[][])  [unwired: 8 in, 2 out]
          n123 = for {
            tunnel: w347 -> [w352] mode=indexing
            shift-right: [w353] -> w348
            shift-left: w349 -> [w354]
            tunnel: w345 -> [w350] mode=indexing
            n124 = call-poly <vilib>:"Write Delimited Spreadsheet.vi"("file path (dialog if empty)"=w352, "1D data"=w350, "append to file? (new file:F)"=TRUE, "error in (no error)"=w354, "delimiter (\\t)"="," ("delimiter (\\t)")) -> ("error out"=w353:errorcluster)  [unwired: 9 in, 1 out]
          }
        }
      }
      frame "Action: Close TDMS File" {
        n125 = Unbundle By Name(w359) -> ("FileHandle.tdms file ref"=w362:refnum<k34>[])
        n126 = flat-sequence {
          tunnel: w359 -> [w370]
          tunnel: [w369] -> w358
          tunnel: w357 -> [_]
          frame #0 {
            n127 = Initialize Array(refnum<k0> refnum, 4 ("dimension size")) -> (w366:refnum<k0>[])
            n128 = Bundle By Name(cluster=w370, "FileHandle.tdms_Initialized"=FALSE, "FileHandle.tdms file ref"=w366) -> (w369:T8)
          }
        }
        n129 = for {
          tunnel: w362 -> [w365] mode=indexing
          shift-right: [w363] -> w360
          shift-left: w361 -> [w364]
          n130 = TDMS Close(8:w364, 11:w365) -> (0:w363:errorcluster)  [unwired: 1 out]
        }
        n131 = call <vilib>:"Clear Errors.vi"("error in (no error)"=w360) -> ("error out"=w357:errorcluster)  [unwired: 5 in, 1 out]
      }
      frame "Action: Close CSV File" {
        n132 = Bundle By Name(cluster=w374, "FileHandle.CSV_Initialized"=FALSE ("FileHandle.tdms_Initialized")) -> (w376:T8)
      }
      frame "Action: ReadData" {
        n133 = Unbundle By Name(w382) -> ("Self Reference"=w381:refnum<class "Log_Engine.lvclass">)
        n134 = call "Read Data.vi"("error in (no error)"=w380, "Log_Engine in"=w381) -> ("error out"=w379:errorcluster, "Log_Engine ReadData"=→"Log_Engine ReadData":T1)  [unwired: 7 in, 1 out]
      }
      frame "Action: Wait" {
        n135 = Scan From String(format string="%d", input string=w386, error in=w385, default 1=u32 0) -> (error out=w384:errorcluster, output 1=w390:u32)  [unwired: 1 in, 2 out]
        n136 = call <userlib>:"Wait (ms)__ogtk.vi"("error in (no error)"=w384, "milliseconds to wait"=w390) -> ("error out"=w388:errorcluster)  [unwired: 8 in, 1 out]
      }
      frame "Action: UpdateSMData" {
        n137 = Match Pattern(string=w400, regular expression=":") -> (before substring=w402:string, after substring=w393:string)  [unwired: 1 in, 2 out]
        n138 = case shown="\"some_data\"" w402 {
          tunnel: w399 -> [_ w409 w424]
          tunnel: w398 -> [_ _ _]
          tunnel: w397 -> [w403 w408 w423]
          tunnel: [w403 w407 w422] -> w396
          tunnel: w395 -> [w404 w406 w421]
          tunnel: [w404 w405 w420] -> w394
          tunnel: w393 -> [_ _ _]
          frame Default {
            # "#NOTE:\noptionally add error here."
          }
          frame "some_data" {
            n139 = disable-structure shown="Disabled" {
              disable-tunnel: w409 -> [w416 _]
              disable-tunnel: w406 -> [w414 w417]
              disable-tunnel: [w413 w417] -> w405
              frame Disabled {
                n140 = Variant To Data(error in=w414, type="", Variant=w416) -> (error out=w413:errorcluster)  [unwired: 1 out]
              }
              frame Enabled {
              }
            }
            n141 = disable-structure shown="Disabled" {
              disable-tunnel: w408 -> [w411 w412]
              disable-tunnel: [w410 w412] -> w407
              frame Disabled {
                n142 = Bundle By Name(cluster=w411) -> (w410:T8)  [unwired: 1 in]
              }
              frame Enabled {
              }
            }
          }
          frame "Settings" {
            n143 = Variant To Data(error in=w421, type=T9 {"Simulation"=FALSE, "TDMS_FolderPath"="", "CSV_FolderPath"="", "TDMS_FileName_Prefix"="", "CSV_FileName_Prefix"="", "TDMS_LogDuration(s)"=0.0, "CSV_LogDuration(s)"=0.0} ("Settings"), Variant=w424) -> (data=w418:T9, error out=w420:errorcluster)
            n144 = Bundle By Name(cluster=w423, "Settings"=w418) -> (w422:T8)
          }
        }
      }
    }
  }
  n145 = while {
    shift-right: [w435] -> _
    shift-left: w5 -> [w434]
    shift-right: [w438] -> w4
    shift-left: w7 -> [w433]
    shift-right: [w437] -> _
    shift-left: w10 -> [w439]
    shift-right: [w432] -> _
    shift-left: _ -> [w431]
    tunnel: w9 -> [w429]
    tunnel: w8 -> [w428]
    tunnel: w2 -> [w427]
    stop <- w436 stop-if-true
    n146 = call <vilib>:"Parse State Queue__JKI_lib_State_Machine.vi"("State Queue"=w439, "Error In (no error)"=w433) -> ("Remaining States"=w441:string, "Current State"=w426:string, "Arguments"=w440:string)  [unwired: 11 in]
    n147 = feedback #1(w427) -> (w425:string)
    n148 = feedback-in #1(w426) -> ()
    n149 = case shown="\"Exit\"" w426 {
      selector: w426 -> [w443 _ _ _ _ _ _ _ _ _ _ _ _ _ _ _ _ _ _ _ _ _ _ _ _ _ _ _]
      tunnel: w441 -> [w447 w462 w468 w476 w576 w589 w597 w602 w606 w611 w620 w627 w632 w640 w649 w661 w688 w694 w705 w710 w721 w730 w743 w760 w771 w780 w789 w798]
      tunnel: w440 -> [_ _ _ _ _ _ _ _ _ _ _ _ _ _ w644 w655 _ _ _ _ w711 _ w737 _ _ _ _ _]
      tunnel: w434 -> [w445 w459 w463 w474 w573 w580 w594 w599 w605 w608 w612 w622 w629 w635 w647 w657 w685 w691 w702 w707 w719 w727 w736 w757 w768 w773 w781 w790]
      tunnel: [w449 errorcluster {"status"=FALSE, "code"=0, "source"=""} ("error out") w466 w473 w574 w586 w590 w600 w603 w609 w618 w623 w630 w636 w645 w658 w686 w692 w703 w708 w712 w722 w739 w753 w764 w775 w783 w792] -> w438
      tunnel: w433 -> [w448 w455 w466 w472 w574 w586 w591 _ w603 w609 w618 w624 w630 w637 w646 w659 w686 w692 w703 w708 w713 w723 w733 w754 w765 w776 w784 w793]
      tunnel: [w446 w461 w467 w475 w575 w588 w596 w602 w606 w610 w619 w626 w631 w639 w648 w660 w687 w693 w704 w709 w720 w729 w742 w759 w770 w779 w788 w797] -> w437
      tunnel: [_ _ TRUE _ _ _ _ _ _ _ _ _ _ _ _ _ _ _ _ _ _ _ _ _ _ _ _ _] -> w436
      tunnel: [w445 w459 w463 w471 w573 w587 w594 w599 w605 w608 w614 w622 w629 w635 w647 w657 w685 w691 w702 w707 w719 w727 w736 w757 w768 w773 w781 w790] -> w435
      tunnel: [w442 w457 w464 w469 w572 w577 w595 w601 w604 w607 w613 w621 w628 w638 w643 w654 w684 w690 w696 w706 w718 w728 w741 w758 w769 w778 w787 w796] -> w432
      tunnel: w431 -> [w442 w457 w464 w469 w572 w577 w595 _ w604 w607 w613 w621 w628 w638 w643 w654 w684 w690 w696 w706 w718 w728 w741 w758 w769 w778 w787 w796]
      tunnel: 200 ("Timeout") -> [_ _ _ w470 _ _ _ _ _ _ _ _ _ _ _ _ _ _ _ _ _ _ _ _ _ _ _ _]
      tunnel: w429 -> [_ _ _ _ _ _ _ _ _ _ _ _ _ _ _ _ _ w689 _ _ _ _ _ _ _ _ _ _]
      tunnel: w428 -> [_ _ _ _ _ _ _ _ _ _ _ _ _ _ _ _ _ _ w695 _ _ _ _ _ _ _ _ _]
      tunnel: w425 -> [_ w454 _ _ _ _ _ _ _ _ _ _ _ _ _ _ _ _ _ _ _ _ _ _ _ _ _ _]
      frame Default {
        w452 = 42 items=["No error", "Argument error", "Memory is full", "Out of zone", "End of file", "File already open", "Generic file I/O error", "File not found", "File permission error", "Disk is full", "Duplicate path", "Too many files open", "System feature not enabled", "Resource file not found", "Cannot add resource", "Resource not found", "Image not found", "Image memory error", "Pen does not exist", "Config type invalid", "Config token not found", "Config parse error", "Config memory error", "Bad external code format", "Bad external code offset", "External code not present", "Null window", "Destroy window error", "Null menu", "Print aborted", "Bad print record", "Print driver error", "Windows error during printing", "Memory error during printing", "Print dialog error", "Generic print error", "Invalid device refnum", "Device not found", "Device parameter error", "Device unit error", "Cannot open device", "Device call aborted", "Generic error", "Cancelled by user", "Object ID too low", "Object ID too high", "Object not in heap", "Unknown heap", "Unknown object (invalid DefProc)", "Unknown object (DefProc not in table)", "Message out of range", "Invalid (null) method", "Unknown message", "Manager call not supported", "Bad address", "Network operation in progress", "Network operation timed out", "Connection is busy", "Network attribute not supported", "Network error", "Address in use", "System out of memory", "Connection aborted", "Connection refused", "Not connected", "Already connected", "Connection closed", "Initialization error (interapplication manager)", "Bad occurrence", "Wait on unbound occurrence handler", "Occurrence queue overflow", "Datalog type conflict", "Unused", "Unrecognized type (interapplication manager)", "Memory corrupt", "Failed to make temporary DLL", "Old CIN version", "Drag socket not found", "Failed to load drop-object", "Failed to register OLE object", "Failed to release OLE object", "Format specifier type mismatch", "Unknown format specifier", "Too few format specifiers", "Too many format specifiers", "Scan failed", "Newer CIN version", "Error converting to variant", "Runtime menu error", "Password tampered", "Variant attribute not found", "Incompatible variant data type", "Event data is not available", "Event Store is not present", "Occurrence is not found", "Event Queue is not created", "Event info is not available", "Refnum passed is NULL", "Error retrieving Class GUID", "Error retrieving CoClass GUID", "Error retrieving TypeLib GUID.", "Bad built application magic bytes.", "Specific driver is different from the specific driver associated with the Logical Name.", "There is no session opened to the class driver.", "Max Error", "MAX - Error with config objects", "MAX - Error loading configuration", "MAX - Group not supported"]
        # "Current State"
        n150 = Format Into String(format string="Software Exception: Unhandled State \"%s\"." ("message"), error in=w448, w443) -> (resulting string=w451:string, error out=w450:errorcluster)  [unwired: 1 in]
        n151 = call <vilib>:"Error Cluster From Error Code.vi"("show call chain? (False)"=TRUE, "error in (no error)"=w450, "error message (\"\")"=w451, "error code (0)"=w452) -> ("error out"=w449:errorcluster)  [unwired: 5 in]
        n152 = call <vilib>:"Add State(s) to Queue__JKI_lib_State_Machine.vi"("State(s) in (\"\")"=w447) -> ("States Out"=w446:string)  [unwired: 14 in]
      }
      frame "Error Handler" {
        n153 = call "General Error Handler - show previous state.vi"("error in (no error)"=w455, "Previous State"=w454, "Loop Select"=enum16{"Event Loop -", "Async Loop -"}."Event Loop -") -> ()  [unwired: 7 in, 2 out]
        n154 = call <vilib>:"Add State(s) to Queue__JKI_lib_State_Machine.vi"("State(s) in Front (\"\")"="/* Post Error States", "State(s) in (\"\")"=w462) -> ("States Out"=w461:string)  [unwired: 13 in]
      }
      frame "Exit" {
        n155 = call <vilib>:"Add State(s) to Queue__JKI_lib_State_Machine.vi"("State(s) in (\"\")"=w468) -> ("States Out"=w467:string)  [unwired: 14 in]
      }
      frame "", "Event Structure", "Idle" {
        n156 = event shown="[5] <Public Events.Log_Engine.AsyncCmd Event>: User Event" {
          selector: w469 -> [_ _ _ _ _ _]
          dyn-events: _ -> [_ _ _ _ _ _]
          timeout: w470 -> [_ _ _ _ _ _]
          tunnel: w476 -> [w480 w485 w491 w494 w501 w521]
          tunnel: [w479 w484 w490 w493 w500 w520] -> w475
          tunnel: w474 -> [w477 w482 w488 w496 w504 w510]
          tunnel: [w478 w483 w489 w497 w505 w518] -> w473
          tunnel: w472 -> [w478 w483 w489 w497 w505 w517]
          tunnel: [w477 w482 w488 w496 w503 w512] -> w471
          event Timeout {
            n157 = event-data() -> ()  [unwired: 1 in, 1 out]
            n158 = call <vilib>:"Add State(s) to Queue__JKI_lib_State_Machine.vi"("State(s) in (\"\")"=w480) -> ("States Out"=w479:string)  [unwired: 14 in]
          }
          event "Exit": Value Change {
            n159 = event-data() -> ()  [unwired: 1 in, 1 out]
            n160 = call <vilib>:"Add State(s) to Queue__JKI_lib_State_Machine.vi"("State(s) in Front (\"\")"="Macro: Exit", "State(s) in (\"\")"=w485) -> ("States Out"=w484:string)  [unwired: 13 in]
          }
          event Panel Close? {
            n161 = event-data() -> ()  [unwired: 1 in, 1 out]
            n162 = event-data("Discard?"=TRUE) -> ()  [unwired: 1 in, 1 out]
            n163 = call <vilib>:"Add State(s) to Queue__JKI_lib_State_Machine.vi"("State(s) in Front (\"\")"="Macro: Exit", "State(s) in (\"\")"=w491) -> ("States Out"=w490:string)  [unwired: 13 in]
          }
          event Menu Selection (User) {
            n164 = event-data() -> ("ItemTag"=w495:string)  [unwired: 1 in, 2 out]
            n165 = case shown="\"False\", Default" w495 {
              tunnel: [""] -> w492
              frame "False", Default {
              }
            }
            n166 = call <vilib>:"Add State(s) to Queue__JKI_lib_State_Machine.vi"("State(s) in Front (\"\")"=w492, "State(s) in (\"\")"=w494) -> ("States Out"=w493:string)  [unwired: 13 in]
          }
          event User Event {
            n167 = event-data() -> ("notifier out"=w502:refnum<notifier>)  [unwired: 1 in]
            n168 = Bundle By Name(cluster=w504, "process sync"=w502) -> (w503:T8)
            n169 = call <vilib>:"Add State(s) to Queue__JKI_lib_State_Machine.vi"("State(s) in Front (\"\")"="Macro: Exit", "State(s) in (\"\")"=w501) -> ("States Out"=w500:string)  [unwired: 13 in]
          }
          event User Event {
            n170 = event-data() -> ("CmdMsg"=w515:string, "vData"=w519:variant)  [unwired: 1 in, 1 out]
            n171 = Unbundle By Name(w510) -> ("Self Reference"=w511:refnum<class "Log_Engine.lvclass">, "Dependency.DAQ_Engine"=w509:refnum<class "DAQ_Engine.lvclass">)
            n172 = call "Get DAQState.vi"("DAQ_Engine in"=w509) -> ("error out"=w508:errorcluster, "DAQState Data"=w507:T21)  [unwired: 8 in, 1 out]
            n173 = call "get async cmd.vi"("error in (no error)"=w517, "Cmd String in"=w515) -> ("error out"=w516:errorcluster, "AsyncCmd"=w514:T2)  [unwired: 8 in]
            n174 = Unbundle(w507) -> ("DAQState"=w506:T22)  [unwired: 1 out]
            n175 = case shown="\"Log_Engine.StopESRLog\"" w514 {
              tunnel: w519 -> [_ w535 w546 w556 w566]
              tunnel: w516 -> [w527 w534 w545 w555 w565]
              tunnel: [w526 w533 w544 w554 w564] -> w518
              tunnel: [_ "Action: Create TDMS File" "Action: Close TDMS File" "Action: Create CSV File" "Action: Close CSV File"] -> w513
              tunnel: w510 -> [w522 w531 w542 w552 w562]
              tunnel: [w522 w530 w542 w552 w562] -> w512
              tunnel: w511 -> [_ _ _ _ _]
              tunnel: w510 -> [_ _ _ _ _]
              tunnel: w508 -> [_ _ _ _ _]
              tunnel: w506 -> [_ _ _ _ _]
              frame Default {
                n176 = call <vilib>:"Build Error Cluster_ModKT .vi"("Prepend String (\"\")"="Invalid Async Cmd" ("Prepend String (\"\")"), "code"=42, "error? (F)"=TRUE, "error in (no error)"=w527) -> ("error out"=w526:errorcluster)  [unwired: 3 in, 1 out]
              }
              frame "Log_Engine.StartLog" {
                n177 = disable-structure shown="Enabled" {
                  disable-tunnel: w535 -> [w540 _]
                  disable-tunnel: w534 -> [w539 w541]
                  disable-tunnel: [w538 w541] -> w533
                  disable-tunnel: [w536 _] -> w528
                  frame Disabled {
                    n178 = Variant To Data(error in=w539, type="", Variant=w540) -> (data=w536:string, error out=w538:errorcluster)
                  }
                  frame Enabled {
                  }
                }
                n179 = To Variant(anything=w528) -> (Variant=w529:variant)
                n180 = Bundle By Name(cluster=w531, "vData"=w529) -> (w530:T8)
              }
              frame "Log_Engine.StopLog" {
                n181 = disable-structure shown="Enabled" {
                  disable-tunnel: w546 -> [w550 _]
                  disable-tunnel: w545 -> [w549 w551]
                  disable-tunnel: [w548 w551] -> w544
                  frame Disabled {
                    n182 = Variant To Data(error in=w549, type="", Variant=w550) -> (error out=w548:errorcluster)  [unwired: 1 out]
                  }
                  frame Enabled {
                  }
                }
              }
              frame "Log_Engine.StartESRLog" {
                n183 = disable-structure shown="Enabled" {
                  disable-tunnel: w556 -> [w560 _]
                  disable-tunnel: w555 -> [w559 w561]
                  disable-tunnel: [w558 w561] -> w554
                  frame Disabled {
                    n184 = Variant To Data(error in=w559, type="", Variant=w560) -> (error out=w558:errorcluster)  [unwired: 1 out]
                  }
                  frame Enabled {
                  }
                }
              }
              frame "Log_Engine.StopESRLog" {
                n185 = disable-structure shown="Enabled" {
                  disable-tunnel: w566 -> [w570 _]
                  disable-tunnel: w565 -> [w569 w571]
                  disable-tunnel: [w568 w571] -> w564
                  frame Disabled {
                    n186 = Variant To Data(error in=w569, type="", Variant=w570) -> (error out=w568:errorcluster)  [unwired: 1 out]
                  }
                  frame Enabled {
                  }
                }
              }
            }
            n187 = call <vilib>:"Add State(s) to Queue__JKI_lib_State_Machine.vi"("State(s) in Front (\"\")"=w513, "State(s) in (\"\")"=w521) -> ("States Out"=w520:string)  [unwired: 13 in]
          }
        }
      }
      frame "---------- Core ----------" {
        n188 = call <vilib>:"Add State(s) to Queue__JKI_lib_State_Machine.vi"("State(s) in (\"\")"=w576) -> ("States Out"=w575:string)  [unwired: 14 in]
      }
      frame "Initialize Core Data" {
        # "originally closed?"
        # "exe?"
        n189 = property class="VI"() -> ("Front Panel.Open"=w585:bool)  [unwired: 2 in, 2 out]
        n190 = property class="App"() -> ("App.Kind"=w584:T19)  [unwired: 2 in, 2 out]
        n191 = control-ref of="Current VI Reference"() -> (w578:refnum<vi>)
        n192 = Not(x=w585) -> (.not. x?=w582:bool)
        n193 = Equal?(x=w584, y=T19."Run Time System" ("Application:Kind")) -> (x = y?=w581:bool)
        n194 = Or(x=w582, y=w581) -> (x .or. y?=w579:bool)
        n195 = Bundle By Name(cluster=w580, "Core.Current VI Reference"=w578, "Core.Close Panel on Exit?"=w579) -> (w587:T8)
        n196 = call <vilib>:"Add State(s) to Queue__JKI_lib_State_Machine.vi"("State(s) in (\"\")"=w589) -> ("States Out"=w588:string)  [unwired: 14 in]
      }
      frame "Process Sync" {
        n197 = Unbundle By Name(w594) -> ("process sync"=w593:refnum<notifier>)
        n198 = Send Notification(notification=TRUE, notifier=w593, error in (no error)=w591) -> (error out=w590:errorcluster)  [unwired: 1 out]
        n199 = call <vilib>:"Add State(s) to Queue__JKI_lib_State_Machine.vi"("State(s) in (\"\")"=w597) -> ("States Out"=w596:string)  [unwired: 14 in]
      }
      frame "DE_Register" {
        n200 = Unbundle By Name(w599) -> ("Public Events"=w598:T11)
        n201 = register-events(w598) -> (reference out=w601:refnum<event-registration>, error out=w600:errorcluster)  [unwired: 2 in]
      }
      frame "DE_Unregister" {
        n202 = Unregister For Events(event registration refnum=w604, error in=w603) -> ()  [unwired: 1 out]
      }
      frame "---------- Data ----------" {
        n203 = call <vilib>:"Add State(s) to Queue__JKI_lib_State_Machine.vi"("State(s) in (\"\")"=w611) -> ("States Out"=w610:string)  [unwired: 14 in]
      }
      frame "Data: Initialize" {
        w615 = T23 {"Current VI Reference"=refnum, "Close Panel on Exit?"=FALSE}  # Core
        w617 = TRUE  # Your Boolean data
        w616 = ""  # Your string data
        n204 = Unbundle By Name(w612) -> ()  [unwired: 1 out]
        n205 = Bundle By Name(cluster=w612, "Core"=w615, "Your Boolean data"=w617, "Your string data"=w616) -> (w614:T8)
        n206 = call <vilib>:"Add State(s) to Queue__JKI_lib_State_Machine.vi"("State(s) in (\"\")"=w620) -> ("States Out"=w619:string)  [unwired: 14 in]
      }
      frame "Data: Cleanup" {
        n207 = Unbundle By Name(w622) -> ("Core.Current VI Reference"=w625:refnum<vi>)
        n208 = Close Reference(reference=w625, error in (no error)=w624) -> (error out=w623:errorcluster)
        n209 = call <vilib>:"Add State(s) to Queue__JKI_lib_State_Machine.vi"("State(s) in (\"\")"=w627) -> ("States Out"=w626:string)  [unwired: 14 in]
      }
      frame "---------- UI ----------" {
        n210 = call <vilib>:"Add State(s) to Queue__JKI_lib_State_Machine.vi"("State(s) in (\"\")"=w632) -> ("States Out"=w631:string)  [unwired: 14 in]
      }
      frame "UI: Initialize" {
        n211 = Unbundle By Name(w635) -> ("Core.Current VI Reference"=w634:refnum<vi>)
        n212 = call <userlib>:"Fit VI window to Largest Dec__ogtk.vi"("error in (no error)"=w637, "VI Ref (calling VI)"=w634) -> ("error out"=w636:errorcluster, "dup VI Ref"=w633:refnum<vi>)  [unwired: 4 in]
        n213 = disable-structure shown="Disabled" {
          disable-tunnel: w633 -> [w642 _]
          frame Disabled {
            n214 = property class="VI"(reference=w642, "Front Panel.Title"="*VI Title*" ("Front Panel Window:Title")) -> ()  [unwired: 1 in, 2 out]
          }
          frame Enabled {
          }
        }
        n215 = call <vilib>:"Add State(s) to Queue__JKI_lib_State_Machine.vi"("State(s) in (\"\")"=w640) -> ("States Out"=w639:string)  [unwired: 14 in]
      }
      frame "UI: Cursor Set" {
        # "Argument"
        n216 = case shown="\"Idle\", Default" w644 {
          tunnel: w646 -> [w651 w653]
          tunnel: [w650 w652] -> w645
          frame "Idle", Default {
            n217 = call <vilib>:"Unset Busy.vi"("error in (no error)"=w651) -> ("error out"=w650:errorcluster)  [unwired: 10 in]
          }
          frame "Busy" {
            n218 = call <vilib>:"Set Busy.vi"("error in (no error)"=w653) -> ("error out"=w652:errorcluster)  [unwired: 9 in, 1 out]
          }
        }
        n219 = call <vilib>:"Add State(s) to Queue__JKI_lib_State_Machine.vi"("State(s) in (\"\")"=w649) -> ("States Out"=w648:string)  [unwired: 14 in]
      }
      frame "UI: Front Panel State" {
        # "Argument"
        n220 = Unbundle By Name(w657) -> ("Core.Current VI Reference"=w656:refnum<vi>)
        n221 = case shown="\"Open\", Default" w655 {
          tunnel: w659 -> [w665 w678]
          tunnel: [w667 w679] -> w658
          tunnel: w656 -> [w666 w676]
          frame "Open", Default {
            n222 = property class="VI"(reference=w666, error in=w665) -> (reference out=w663:refnum<vi>, error out=w664:errorcluster, "Front Panel.Open"=w662:bool)
            n223 = case shown="False" w662 {
              tunnel: [w670 w673] -> w667
              tunnel: w664 -> [w669 w673]
              tunnel: w663 -> [w668 _]
              frame False {
                n224 = invoke class="VI" method="FP.Open"(reference=w668, error in=w669, "Activate"=TRUE, "State"=T20."Standard") -> (error out=w670:errorcluster)  [unwired: 1 in, 4 out]
              }
              frame True {
              }
            }
          }
          frame "Close" {
            n225 = property class="VI"(reference=w676, error in=w678) -> (reference out=w675:refnum<vi>, error out=w677:errorcluster, "Front Panel.Open"=w674:bool)
            n226 = case shown="True" w674 {
              tunnel: [w680 w683] -> w679
              tunnel: w677 -> [w680 w682]
              tunnel: w675 -> [_ w681]
              frame False {
              }
              frame True {
                n227 = invoke class="VI" method="FP.Close"(reference=w681, error in=w682) -> (error out=w683:errorcluster)  [unwired: 1 in, 2 out]
              }
            }
          }
        }
        n228 = call <vilib>:"Add State(s) to Queue__JKI_lib_State_Machine.vi"("State(s) in (\"\")"=w661) -> ("States Out"=w660:string)  [unwired: 14 in]
      }
      frame "---------- Macro ----------" {
        n229 = call <vilib>:"Add State(s) to Queue__JKI_lib_State_Machine.vi"("State(s) in (\"\")"=w688) -> ("States Out"=w687:string)  [unwired: 14 in]
      }
      frame "Macro: Initialize" {
        n230 = call <vilib>:"Add State(s) to Queue__JKI_lib_State_Machine.vi"("State(s) in Front (\"\")"=w689, "State(s) in (\"\")"=w694) -> ("States Out"=w693:string)  [unwired: 13 in]
      }
      frame "Macro: Exit" {
        n231 = Unbundle By Name(w702) -> ("Core.Close Panel on Exit?"=w701:bool)
        n232 = Select(t="UI: Front Panel State >> Close", s=w701, f="") -> (s? t:f=w698:string)
        n233 = call <vilib>:"Add State(s) to Queue__JKI_lib_State_Machine.vi"("State(s) in (\"\")"=w698, "State(s) at Back (\"\")"=w695) -> ("States Out"=w697:string)  [unwired: 13 in]
        n234 = call <vilib>:"Add State(s) to Queue__JKI_lib_State_Machine.vi"("State(s) in Front (\"\")"=w697, "State(s) in (\"\")"=w705) -> ("States Out"=w704:string)  [unwired: 13 in]
      }
      frame "---------- Action ----------" {
        n235 = call <vilib>:"Add State(s) to Queue__JKI_lib_State_Machine.vi"("State(s) in (\"\")"=w710) -> ("States Out"=w709:string)  [unwired: 14 in]
      }
      frame "Action: Wait" {
        n236 = Scan From String(format string="%d", input string=w711, error in=w713, default 1=u32 0) -> (error out=w717:errorcluster, output 1=w716:u32)  [unwired: 1 in, 2 out]
        n237 = call <userlib>:"Wait (ms)__ogtk.vi"("error in (no error)"=w717, "milliseconds to wait"=w716) -> ("error out"=w712:errorcluster)  [unwired: 8 in, 1 out]
        n238 = call <vilib>:"Add State(s) to Queue__JKI_lib_State_Machine.vi"("State(s) in (\"\")"=w721) -> ("States Out"=w720:string)  [unwired: 14 in]
      }
      frame "Action: Terminate AsyncLoop" {
        n239 = Unbundle By Name(w727) -> ("SMQ"=w726:refnum<queue>)
        n240 = Flush Queue(queue=w726) -> (queue out=w725:refnum<queue>)  [unwired: 1 in, 2 out]
        n241 = call <vilib>:"Add State to Queue with vData.vi"("queue in"=w725, "state in"="Macro: Exit", "error in"=w723) -> ("error out"=w722:errorcluster)  [unwired: 9 in, 3 out]
        n242 = call <vilib>:"Add State(s) to Queue__JKI_lib_State_Machine.vi"("State(s) in (\"\")"=w730) -> ("States Out"=w729:string)  [unwired: 14 in]
      }
      frame "Action: UpdateSMData" {
        n243 = Unbundle By Name(w736) -> ("SMQ"=w740:refnum<queue>)
        n244 = Format Into String(format string="Action: UpdateSMData:%s" ("state in"), error in=w733, w737) -> (resulting string=w732:string, error out=w734:errorcluster)  [unwired: 1 in]
        n245 = case shown="\"Settings\"" w737 {
          tunnel: w736 -> [_ w749]
          tunnel: [variant ("Variant") w747] -> w735
          tunnel: w732 -> [_ w746]
          tunnel: ["" w746] -> w731
          frame "False", Default {
          }
          frame "Settings" {
            n246 = Unbundle By Name(w749) -> ("Settings"=w748:T9)
            n247 = To Variant(anything=w748) -> (Variant=w747:variant)
          }
        }
        n248 = call <vilib>:"Add State to Queue with vData.vi"("queue in"=w740, "state in"=w731, "vData (\"\")"=w735, "error in"=w734) -> ("error out"=w739:errorcluster)  [unwired: 8 in, 3 out]
        n249 = call <vilib>:"Add State(s) to Queue__JKI_lib_State_Machine.vi"("State(s) in (\"\")"=w743) -> ("States Out"=w742:string)  [unwired: 14 in]
      }
      frame "Action: Close TDMS File" {
        n250 = Unbundle By Name(w757) -> ("SMQ"=w756:refnum<queue>)
        n251 = Flush Queue(queue=w756) -> (queue out=w752:refnum<queue>)  [unwired: 1 in, 2 out]
        n252 = call "ReverseStringLines.vi"("Lines in"="Action: Close TDMS File\nAction: Set TDMS Logging State >> OFF" ("state in")) -> ("Reversed Lines out"=w750:string)  [unwired: 4 in]
        n253 = call-poly <vilib>:"Polymorphic - Add States(s) To Queue.vi"("queue in"=w752, "mode (back)"=enum16{"back", "front"}."front", "states in"=w750, "error in"=w754) -> ("error out"=w753:errorcluster)  [unwired: 9 in, 2 out]
        n254 = call <vilib>:"Add State(s) to Queue__JKI_lib_State_Machine.vi"("State(s) in (\"\")"=w760) -> ("States Out"=w759:string)  [unwired: 14 in]
      }
      frame "Action: Close CSV File" {
        n255 = Unbundle By Name(w768) -> ("SMQ"=w767:refnum<queue>)
        n256 = Flush Queue(queue=w767) -> (queue out=w763:refnum<queue>)  [unwired: 1 in, 2 out]
        n257 = call "ReverseStringLines.vi"("Lines in"="Action: Close CSV File\nAction: Set CSV Logging State >> OFF" ("state in")) -> ("Reversed Lines out"=w761:string)  [unwired: 4 in]
        n258 = call-poly <vilib>:"Polymorphic - Add States(s) To Queue.vi"("queue in"=w763, "mode (back)"=enum16{"back", "front"}."front", "states in"=w761, "error in"=w765) -> ("error out"=w764:errorcluster)  [unwired: 9 in, 2 out]
        n259 = call <vilib>:"Add State(s) to Queue__JKI_lib_State_Machine.vi"("State(s) in (\"\")"=w771) -> ("States Out"=w770:string)  [unwired: 14 in]
      }
      frame "Action: Create TDMS File" {
        n260 = Unbundle By Name(w773) -> ("SMQ"=w772:refnum<queue>, "vData"=w774:variant)
        n261 = call-poly <vilib>:"Polymorphic - Add States(s) To Queue.vi"("queue in"=w772, "states in"="Action: Create TDMS File\nAction: Set TDMS Logging State >> ON" ("state in"), "vData (\"\")"=w774, "error in"=w776) -> ("error out"=w775:errorcluster)  [unwired: 9 in, 2 out]
        n262 = call <vilib>:"Add State(s) to Queue__JKI_lib_State_Machine.vi"("State(s) in (\"\")"=w780) -> ("States Out"=w779:string)  [unwired: 14 in]
      }
      frame "Action: Create CSV File" {
        n263 = Unbundle By Name(w781) -> ("SMQ"=w786:refnum<queue>, "vData"=w782:variant)
        n264 = call-poly <vilib>:"Polymorphic - Add States(s) To Queue.vi"("queue in"=w786, "states in"="Action: Create CSV File\nAction: Set CSV Logging State >> ON" ("state in"), "vData (\"\")"=w782, "error in"=w784) -> ("error out"=w783:errorcluster)  [unwired: 9 in, 2 out]
        n265 = call <vilib>:"Add State(s) to Queue__JKI_lib_State_Machine.vi"("State(s) in (\"\")"=w789) -> ("States Out"=w788:string)  [unwired: 14 in]
      }
      frame "Action: Close Logging Loop" {
        n266 = Unbundle By Name(w790) -> ("SMQ"=w795:refnum<queue>, "vData"=w791:variant)
        n267 = call <vilib>:"Add State to Queue with vData.vi"("queue in"=w795, "state in"="Exit", "vData (\"\")"=w791, "error in"=w793) -> ("error out"=w792:errorcluster)  [unwired: 8 in, 3 out]
        n268 = call <vilib>:"Add State(s) to Queue__JKI_lib_State_Machine.vi"("State(s) in (\"\")"=w798) -> ("States Out"=w797:string)  [unwired: 14 in]
      }
    }
  }
  n269 = Merge Errors(w4, w3) -> ()  [unwired: 1 out]
